vi "Exit Check Dialog.vi"(11 "Monitor":i16) -> (3 "Exit?":bool)   [LabVIEW 2017, in "Debug Server.lvclass"]
doc: "Simple dialog to confirm with user whether or not Debug Server application server should shut down."
uses:
  Debug Server.lvclass
panel:
  in  "Cancel":bool
  in  "OK":bool
  in  "Title":string="Message Logs are still open.\n \nExit anyway?"
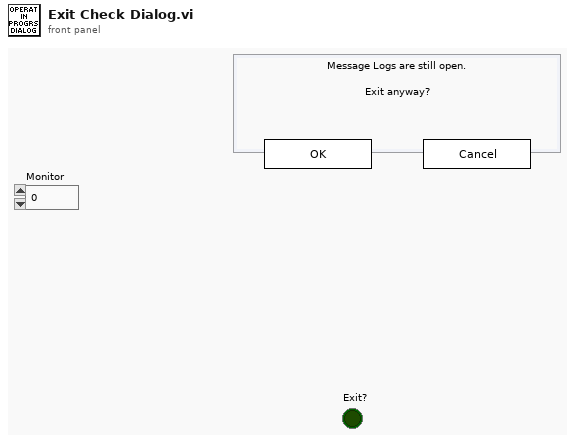
[diagram p1: front panel]
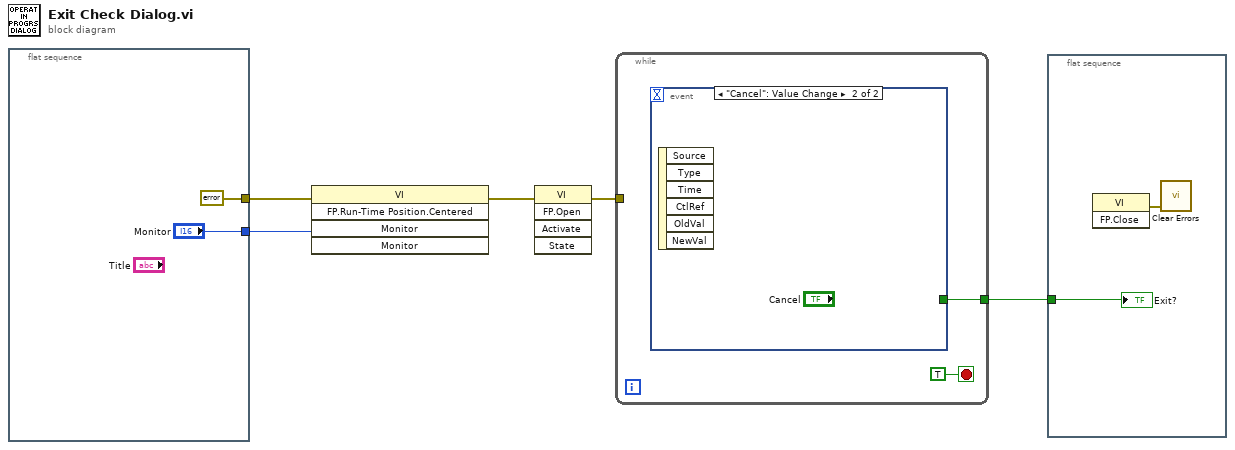
[diagram p0: block diagram]
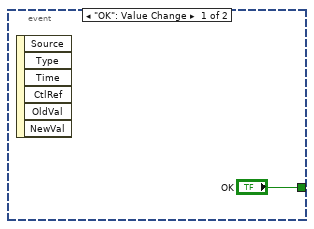
[diagram p2: hidden frame]
diagram:
  n1 = flat-sequence {
    tunnel: [errorcluster {"status"=FALSE, "code"=0, "source"=""} ("error out")] -> w3
    tunnel: ["Monitor"] -> w2
    frame #0 {
    }
  }
  n2 = invoke class="VI" method="FP.Run-Time Position.Centered"(error in=w3, "Monitor"=w2) -> (error out=w5:errorcluster)  [unwired: 3 in, 4 out]
  n3 = invoke class="VI" method="FP.Open"(error in=w5) -> (error out=w4:errorcluster)  [unwired: 4 in, 4 out]
  n4 = while {
    tunnel: w4 -> [_]
    tunnel: [w8] -> w1
    stop <- TRUE stop-if-true
    n5 = event shown="[1] \"Cancel\": Value Change" {
      selector: _ -> [_ _]
      dyn-events: _ -> [_ _]
      timeout: _ -> [_ _]
      tunnel: ["OK" _] -> w8
      event "OK": Value Change {
        n6 = event-data() -> ()  [unwired: 1 in, 6 out]
      }
      event "Cancel": Value Change {
        n7 = event-data() -> ()  [unwired: 1 in, 6 out]
      }
    }
  }
  n8 = flat-sequence {
    tunnel: w1 -> [w11]
    frame #0 {
      n9 = invoke class="VI" method="FP.Close"() -> (error out=w12:errorcluster)  [unwired: 3 in, 2 out]
      n10 = call <vilib>:"Clear Errors.vi"("error in (no error)"=w12) -> ()  [unwired: 5 in, 2 out]
      "Exit?" <- w11
    }
  }
